vi "get glyphArray.vi"(8 "error in (no error)":errorcluster, 11 "xceRootNode in":refnum<class "xceRootNode.lvclass">) -> (0 "error out":errorcluster, 2 "glyphArray":string[](array[string]), 3 "xceRootNode out":refnum<class "xceRootNode.lvclass">)   [LabVIEW 2013, in "xceRootNode.lvclass"]
uses:
  xceRootNode.lvclass
  xceRootNode.lvclass/xceRootNode.ctl
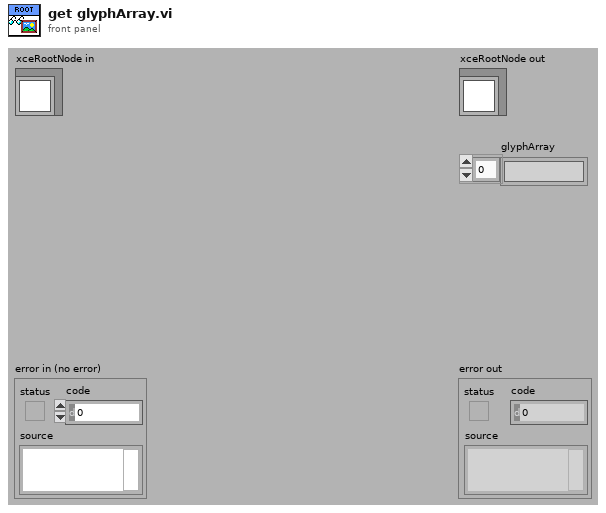
[diagram p1: front panel]
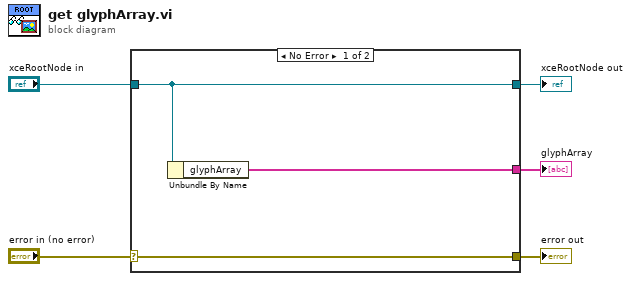
[diagram p0: block diagram]
diagram:
  n1 = case shown="No Error" "error in (no error)" {
    selector: "error in (no error)" -> [w8 w9]
    tunnel: [w8 w9] -> w4
    tunnel: [w7 w10] -> w2
    tunnel: "xceRootNode in" -> [w7 w10]
    tunnel: [w6 _] -> w1
    frame No Error {
      n2 = Unbundle By Name(w7) -> ("glyphArray"=w6:string[])
    }
    frame Error {
    }
  }
  "error out" <- w4
  "xceRootNode out" <- w2
  "glyphArray" <- w1
